vi "2-input NAND.vi"(10 "Obtained Expression":string, 11 "Input List":string[](array[string])) -> (1 "O/p = I/p":string, 2 "NAND ?":bool, 3 "Logic Exp":string)   [LabVIEW 2014]
doc: "This VI is used to compare the obtained logic with the logic of NAND gate."
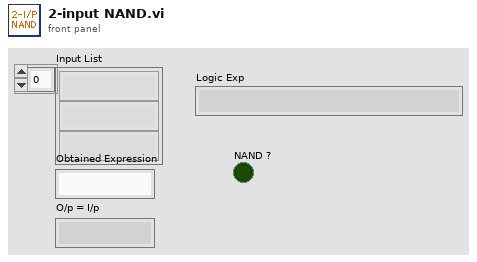
[diagram p1: front panel]
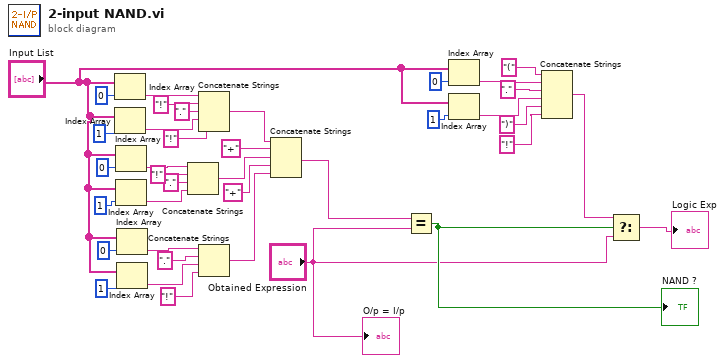
[diagram p0: block diagram]
diagram:
  n1 = Index Array(array="Input List", index=0) -> (element=w20:string)
  n2 = Index Array(array="Input List", index=1) -> (element=w23:string)
  n3 = Index Array(array="Input List", index=0) -> (element=w29:string)
  n4 = Index Array(array="Input List", index=1) -> (element=w26:string)
  n5 = Index Array(array="Input List", index=0) -> (element=w35:string)
  n6 = Index Array(array="Input List", index=1) -> (element=w37:string)
  n7 = Concatenate Strings(w29, "!" ("t"), "." ("string"), w26) -> (w31:string)
  n8 = Concatenate Strings(w20, "!" ("t"), "." ("string"), w23, "!" ("t")) -> (w24:string)
  n9 = Concatenate Strings(w35, "." ("string"), w37, "!" ("string")) -> (w38:string)
  n10 = Concatenate Strings(w24, "+" ("string"), w31, "+" ("string"), w38) -> (w15:string)
  n11 = Equal?(x=w15, y="Obtained Expression") -> (x = y?=w14:bool)
  "NAND ?" <- w14
  n12 = Index Array(array="Input List", index=0) -> (element=w10:string)
  n13 = Index Array(array="Input List", index=1) -> (element=w8:string)
  n14 = Concatenate Strings("(" ("string"), w10, "." ("string"), w8, ")" ("string"), "!" ("string")) -> (w4:string)
  n15 = Select(t=w4, s=w14, f="Obtained Expression") -> (s? t:f=→"Logic Exp":string)
  "O/p = I/p" <- "Obtained Expression"
